vi "Write State Refnum.vi"(8 "error in (no error)":errorcluster, 10 "State Refnum":refnum<vi>, 11 "Data Logger in":refnum<class "Data Logger.lvclass">) -> (0 "error out":errorcluster, 3 "Data Logger out":refnum<class "Data Logger.lvclass">)   [LabVIEW 2013, in "Data Logger.lvlib" / "Data Logger.lvclass"]
uses:
  Data Logger.lvclass
  Display Panel/Abstract Display/Control 1.ctl
  Data Logger.lvclass/Data Logger.ctl
  Display Panel/Abstract Display/Abstract Display.lvclass
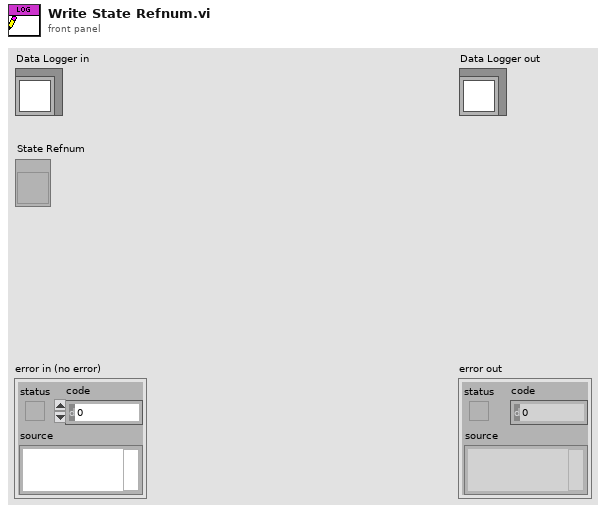
[diagram p1: front panel]
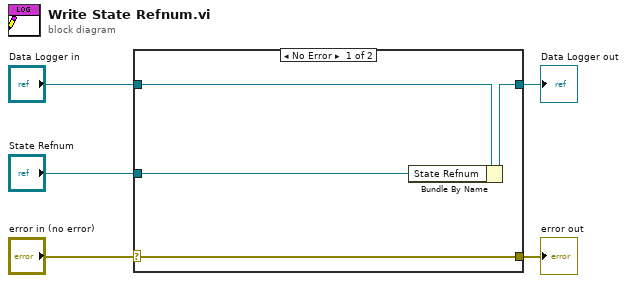
[diagram p0: block diagram]
diagram:
  n1 = case shown="No Error" "error in (no error)" {
    selector: "error in (no error)" -> [w9 w10]
    tunnel: [w9 w10] -> w4
    tunnel: [w7 w11] -> w2
    tunnel: "Data Logger in" -> [w8 w11]
    tunnel: "State Refnum" -> [w6 _]
    frame No Error {
      n2 = Bundle By Name(cluster=w8, "State Refnum"=w6) -> (w7:refnum<class "Data Logger.lvclass">)
    }
    frame Error {
    }
  }
  "error out" <- w4
  "Data Logger out" <- w2
